vi "WPI_SPIRead.vi"(8 "error in (no error)":errorcluster, 10 "Num to Read":i32, 11 "SPIDevRef":T1) -> (0 "error out":errorcluster, 2 "Received Data":u8[](array[numeric]), 3 "SPIDevRef":T1)   [LabVIEW 2017]
doc: "Reads data from the slave device.\n\nThis software is licensed. Open the labview\\readme\\WPI Robotics Library Open Source License.txt file for more information."
uses:
  <vilib>/Rock Robotics/WPI/SPI/WPI_SPIDevRef.ctl
  <vilib>/Rock Robotics/SystemInterfaces/spilib/spi_bus.ctl
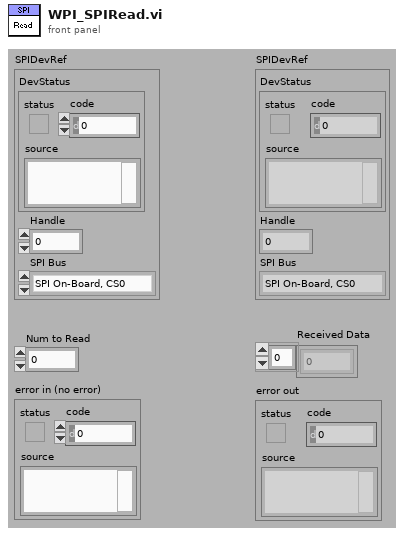
[diagram p1: front panel]
types:
  T1 = typedef "WPI_SPIDevRef.ctl" = cluster{"DevStatus":errorcluster, "Handle":i32, "SPI Bus":T2}
  T2 = typedef "spi_bus.ctl" = enum16{"SPI On-Board, CS0", "SPI On-Board, CS1", "SPI On-Board, CS2", "SPI On-Board, CS3", "SPI MXP", "Invalid"}
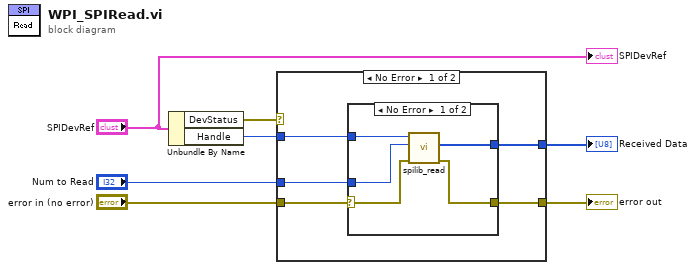
[diagram p0: block diagram]
diagram:
  n1 = Unbundle By Name("SPIDevRef") -> ("DevStatus"=w6:errorcluster, "Handle"=w4:i32)
  n2 = case shown="No Error" w6 {
    selector: w6 -> [_ w19]
    tunnel: "error in (no error)" -> [w12 _]
    tunnel: [w11 w19] -> w5
    tunnel: w4 -> [w10 _]
    tunnel: "Num to Read" -> [w9 _]
    tunnel: [w8 _] -> w2
    frame No Error {
      n3 = case shown="No Error" w12 {
        selector: w12 -> [w16 w18]
        tunnel: [w13 w18] -> w11
        tunnel: w10 -> [w17 _]
        tunnel: w9 -> [w15 _]
        tunnel: [w14 _] -> w8
        frame No Error {
          n4 = call <vilib>:"spilib_read.vi"("error in (no error)"=w16, "recv_size"=w15, "handle"=w17) -> ("error out"=w13:errorcluster, "recv_buf"=w14:i8[])  [unwired: 6 in, 1 out]
        }
        frame Error {
        }
      }
    }
    frame Error {
    }
  }
  "error out" <- w5
  "Received Data" <- w2
  "SPIDevRef" <- "SPIDevRef"
